vi "Feed.vi"(8 "error in (no error)":errorcluster, 9 "W/R":enum16{"Write", "Read"}(ring), 10 "Feed":u32, 11 "Motor Base in":refnum<class "Motor Base.lvclass">) -> (0 "error out":errorcluster, 2 "Data":u32, 3 "Motor Base out":refnum<class "Motor Base.lvclass">)   [LabVIEW 2016, in "Motor Base.lvlib" / "Motor Base.lvclass"]
uses:
  Motor Base.lvclass
  Data Type.ctl
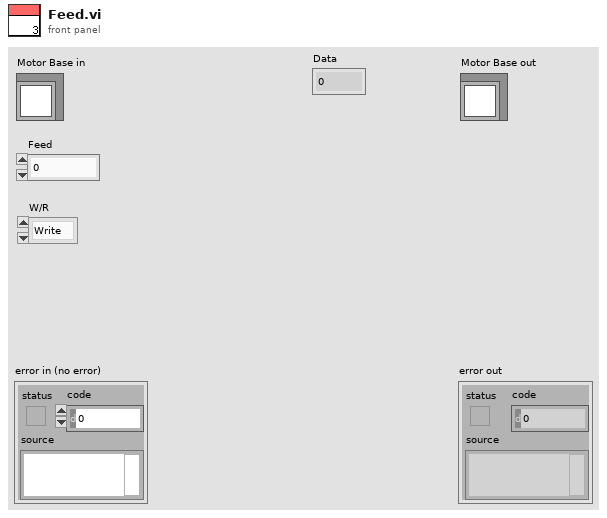
[diagram p1: front panel]
types:
  T1 = typedef "Motor Base.lvlib/Motor Base.lvclass/Data Type.ctl" = enum16{"BOOL", "I16", "I32", "I8", "OS", "U16", "U32", "U8", "VS"}
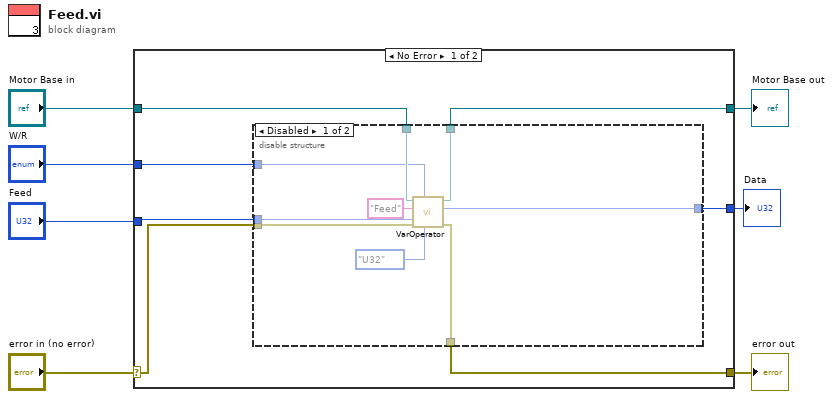
[diagram p0: block diagram]
diagram:
  n1 = case shown="No Error" "error in (no error)" {
    selector: "error in (no error)" -> [w12 w28]
    tunnel: [w11 w28] -> w6
    tunnel: [w13 w27] -> w4
    tunnel: "Motor Base in" -> [w14 w27]
    tunnel: "Feed" -> [w10 _]
    tunnel: [w9 _] -> w2
    tunnel: "W/R" -> [w8 _]
    frame No Error {
      n2 = disable-structure shown="Disabled" {
        disable-tunnel: w14 -> [w23 w26]
        disable-tunnel: [w22 w26] -> w13
        disable-tunnel: w12 -> [w20 w24]
        disable-tunnel: [w19 w24] -> w11
        disable-tunnel: w10 -> [w18 w25]
        disable-tunnel: [w17 w25] -> w9
        disable-tunnel: w8 -> [w15 _]
        frame Disabled {
          n3 = call-dynamic "VarOperator.vi"("Data Type"=Data_Type."U32", "ro/w/r"=w15, "error in"=w20, "Data"=w18, "PDO Name"="Feed", "Motor Base in"=w23) -> ("error out"=w19:errorcluster, "Data"=w17:i64, "Motor Base out"=w22:refnum<class "Motor Base.lvclass">)  [unwired: 1 in, 2 out]
        }
        frame Enabled {
        }
      }
    }
    frame Error {
    }
  }
  "error out" <- w6
  "Motor Base out" <- w4
  "Data" <- w2
